vi "Initialize StartupBehavior Attribute.vi"(7 "Attribute.StartupBehavior in":refnum<class "Attribute.StartupBehavior.lvclass">, 11 "Behavior (Immediate)":T1) -> (3 "Attribute.StartupBehavior":refnum<class "Attribute.StartupBehavior.lvclass">)   [LabVIEW 2021, in "smo.lvlib" / "Attribute.StartupBehavior.lvclass"]
uses:
  Attribute.StartupBehavior.lvclass
  Attribute.StartupBehavior.lvclass/Attribute.StartupBehavior.ctl
  Definitions/def.SMO/Scope -- Enum.ctl
  Definitions/def.SMO/def.SMO.lvclass
  Attribute/Attribute.lvclass
  C:/Repositories/SMO/src/Support/Attribute/Attribute.lvclass
  ProcessStartupBehavior.ctl
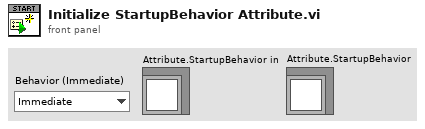
[diagram p1: front panel]
types:
  T1 = typedef "smo.lvlib/Attribute.StartupBehavior.lvclass/ProcessStartupBehavior.ctl" = enum16{"Immediate", "First Call", "Never"}
  T2 = typedef "smo.lvlib/def.SMO.lvclass/Scope -- Enum.ctl" = enum16{"Public", "Protected", "Private"}
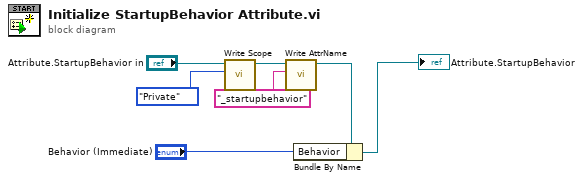
[diagram p0: block diagram]
diagram:
  n1 = call "Write Scope.vi"("Scope"=Scope_--_Enum."Private", "Attribute in"="Attribute.StartupBehavior in") -> ("Attribute out"=w5:refnum<class "Attribute.StartupBehavior.lvclass">)  [unwired: 9 in]
  n2 = call "Write AttrName.vi"("Attribute Name"="_startupbehavior", "Attribute in"=w5) -> ("Attribute out"=w4:refnum<class "Attribute.StartupBehavior.lvclass">)  [unwired: 9 in]
  n3 = Bundle By Name(cluster=w4, "Behavior"="Behavior (Immediate)") -> (→"Attribute.StartupBehavior":refnum<class "Attribute.StartupBehavior.lvclass">)
